vi "test_spline_fft.vi"() -> ()   [LabVIEW 2009]
doc: "Copyright (C) 2009, Stepan A. Baranov\nweb: http://www.OCTLab.org/\nemail: stepan@baranov.su"
uses:
  <vilib>/Analysis/4window.llb/Hanning Window (DBL).vi
  <vilib>/Analysis/NI_AALPro.lvlib
  OCTLib.dll
panel:
  out "error out":errorcluster
  out "Im part":dbl[](array[numeric])
  out "Re part":dbl[](array[numeric])
  out "Phase A-scan":dbl[](array[numeric])
  out "Intensity A-scan":dbl[](array[numeric])
  out "Im":dbl[](array[numeric])
  out "Re":dbl[](array[numeric])
  out "phase":dbl[](array[numeric])
  out "intensity":dbl[](array[numeric])
  out "time for FFT":u32
  in  "RSM_STAT?":bool=TRUE
  in  "stop":bool
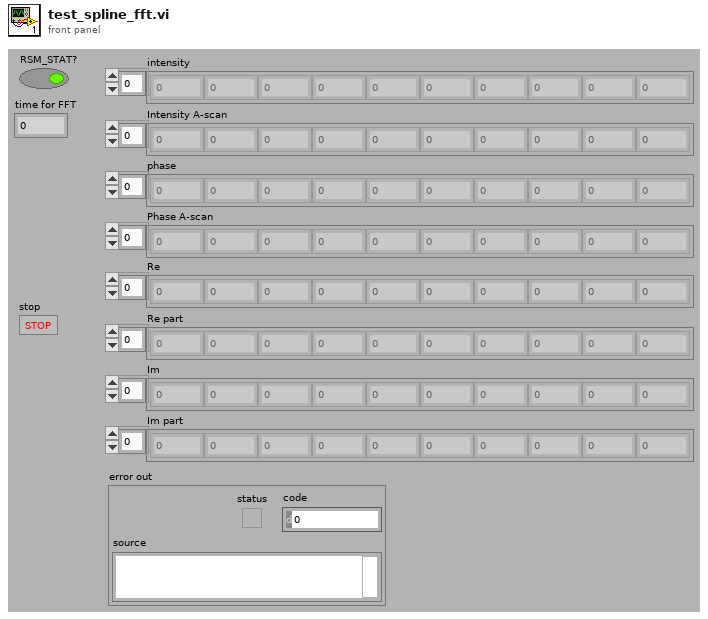
[diagram p1: front panel]
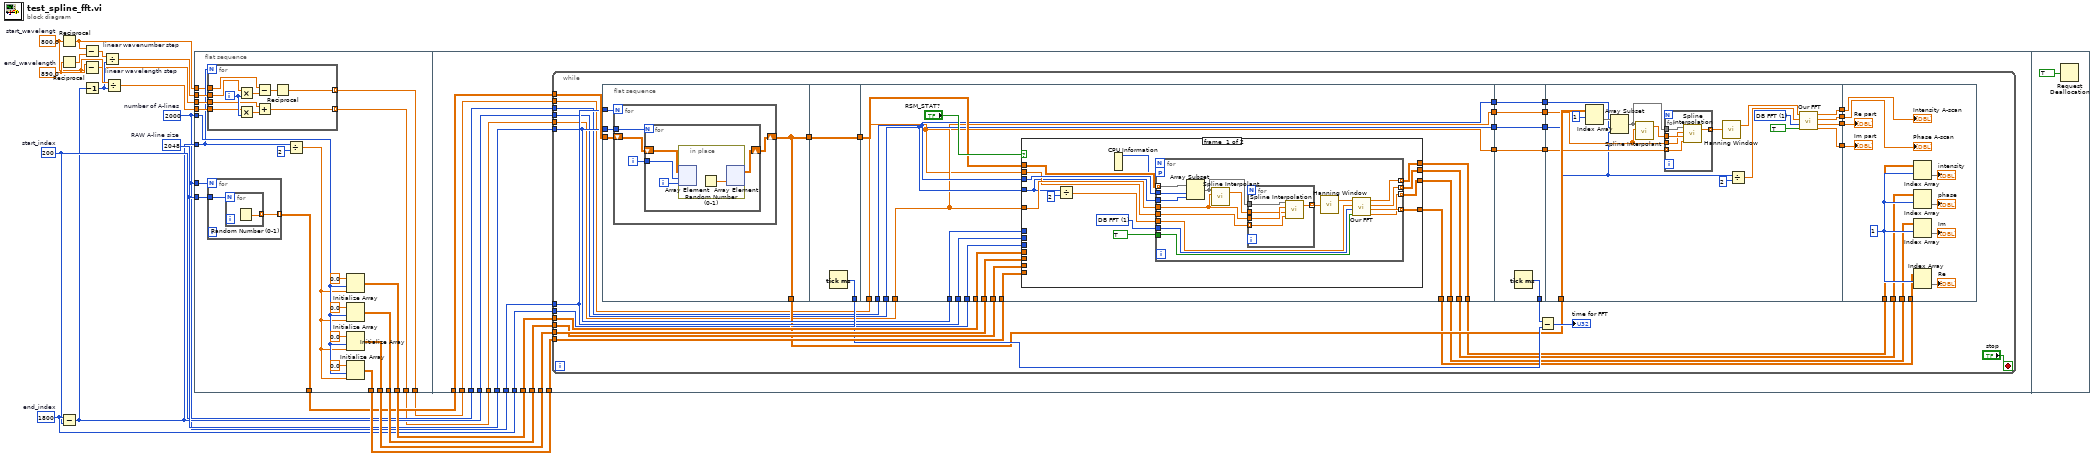
[diagram p0: block diagram]
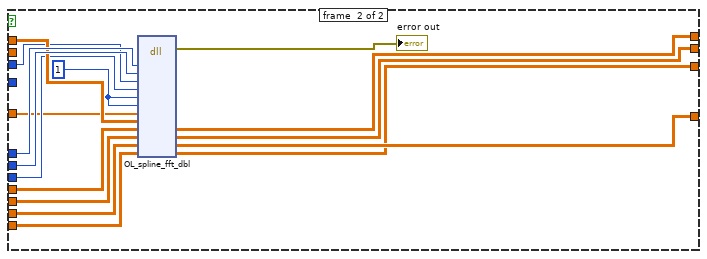
[diagram p2: hidden frame]
diagram:
  w1 = 800.0  # start_wavelengt
  w9 = 890.0  # end_wavelength
  w15 = 1800  # end_index
  w8 = 200  # start_index
  w4 = 2000  # number of A-lines
  w16 = 2048  # RAW A-line size
  n1 = Reciprocal(x=w1) -> (1/x=w2:dbl)
  n2 = Reciprocal(x=w9) -> (1/x=w3:dbl)
  n3 = Subtract(x=w15, y=w8) -> (x-y=w7:i32)
  n4 = Subtract(x=w2, y=w3) -> (x-y=w13:dbl)
  n5 = Subtract(x=w9, y=w1) -> (x-y=w14:dbl)
  n6 = Decrement(x=w7) -> (x-1=w12:i32)
  n7 = Divide "linear wavenumber step"(x=w13, y=w12) -> (x/y=w11:dbl)
  n8 = Divide "linear wavelength step"(x=w14, y=w12) -> (x/y=w10:dbl)
  n9 = flat-sequence {
    tunnel: w16 -> [w42]
    tunnel: w4 -> [w41]
    tunnel: w4 -> [w36]
    tunnel: [w35] -> w21
    tunnel: [w34] -> w20
    tunnel: [w33] -> w19
    tunnel: [w32] -> w18
    tunnel: [w31] -> w17
    tunnel: w7 -> [w26]
    tunnel: w11 -> [w30]
    tunnel: w10 -> [w29]
    tunnel: w1 -> [w28]
    tunnel: [w22] -> w6
    tunnel: [w27] -> w5
    tunnel: w2 -> [w23]
    tunnel: w4 -> [w67]
    tunnel: w16 -> [w66]
    tunnel: w21 -> [w65]
    tunnel: w20 -> [w64]
    tunnel: w19 -> [w63]
    tunnel: w18 -> [w62]
    tunnel: w17 -> [w61]
    tunnel: w8 -> [w60]
    tunnel: w15 -> [w59]
    tunnel: w7 -> [w58]
    tunnel: w6 -> [w57]
    tunnel: w5 -> [w56]
    frame #0 {
      n10 = for {
        N: w26 -> [_]
        tunnel: w30 -> [w52]
        tunnel: [w44] -> w27 mode=indexing
        tunnel: w29 -> [w49]
        tunnel: w28 -> [w48]
        tunnel: [w43] -> w22 mode=indexing
        tunnel: w23 -> [w46]
        i -> [w50]
        n11 = Multiply(x=w52, y=w50) -> (x*y=w51:dbl)
        n12 = Multiply(x=w49, y=w50) -> (x*y=w47:dbl)
        n13 = Subtract(x=w46, y=w51) -> (x-y=w45:dbl)
        n14 = Add(x=w48, y=w47) -> (x+y=w43:dbl)
        n15 = Reciprocal(x=w45) -> (1/x=w44:dbl)
      }
      n16 = for {
        N: w41 -> [_]
        tunnel: [w54] -> w31 mode=indexing
        tunnel: w42 -> [w53]
        n17 = for {
          N: w53 -> [_]
          tunnel: [w55] -> w54 mode=indexing
          n18 = Random Number (0-1)() -> (number: 0 to 1=w55:dbl)
        }
      }
      n19 = Divide(x=w26, y=2) -> (x/y=w24:dbl)
      n20 = Initialize Array(0.0 ("element"), w36, w24) -> (w34:dbl[][])
      n21 = Initialize Array(0.0 ("element"), w36, w24) -> (w33:dbl[][])
      n22 = Initialize Array(0.0 ("element"), w36, w24) -> (w35:dbl[][])
      n23 = Initialize Array(0.0 ("element"), w36, w24) -> (w32:dbl[][])
    }
    frame #1 {
      n24 = while {
        tunnel: w61 -> [w101]
        tunnel: w67 -> [w93]
        tunnel: w66 -> [w92]
        tunnel: w65 -> [w100]
        tunnel: w64 -> [w99]
        tunnel: w63 -> [w98]
        tunnel: w62 -> [w97]
        tunnel: w60 -> [w80]
        tunnel: w59 -> [w79]
        tunnel: w58 -> [w78]
        tunnel: w57 -> [w77]
        tunnel: w56 -> [w76]
        stop <- "stop" stop-if-true
        n25 = flat-sequence {
          tunnel: w101 -> [w106]
          tunnel: w93 -> [w105]
          tunnel: w92 -> [w104]
          tunnel: [w103] -> w91
          tunnel: [w103] -> w81
          tunnel: [w117] -> w96
          tunnel: [w116] -> w82
          tunnel: w81 -> [w116]
          tunnel: w100 -> [w133]
          tunnel: w99 -> [w132]
          tunnel: w98 -> [w131]
          tunnel: w97 -> [w130]
          tunnel: w92 -> [w129]
          tunnel: w93 -> [w128]
          tunnel: [w127] -> w86
          tunnel: [w126] -> w85
          tunnel: [w125] -> w84
          tunnel: [w124] -> w83
          tunnel: w82 -> [w123]
          tunnel: w80 -> [w121]
          tunnel: w79 -> [w122]
          tunnel: w78 -> [w120]
          tunnel: w77 -> [w119]
          tunnel: w76 -> [w118]
          tunnel: [w121] -> w74
          tunnel: [w120] -> w72
          tunnel: [w119] -> w71
          tunnel: [w118] -> w68
          tunnel: [w190] -> w94
          tunnel: [w189] -> w75
          tunnel: w74 -> [w189]
          tunnel: [w188] -> w73
          tunnel: w72 -> [w188]
          tunnel: w71 -> [w187]
          tunnel: [w187] -> w70
          tunnel: [w186] -> w69
          tunnel: w68 -> [w186]
          tunnel: w91 -> [w209]
          tunnel: [w204] -> w90
          tunnel: [w203] -> w89
          tunnel: [w202] -> w88
          tunnel: [w201] -> w87
          tunnel: w75 -> [w198]
          tunnel: w73 -> [w193]
          tunnel: w70 -> [w196]
          tunnel: w69 -> [w195]
          tunnel: w90 -> [w227]
          tunnel: w89 -> [w226]
          tunnel: w88 -> [w225]
          tunnel: w87 -> [w224]
          tunnel: w86 -> [w222]
          tunnel: w85 -> [w220]
          tunnel: w84 -> [w218]
          tunnel: w83 -> [w216]
          frame #0 {
            n26 = for {
              N: w105 -> [_]
              shift-right: [w108] -> w103
              shift-left: w106 -> [w109]
              tunnel: w104 -> [w110]
              i -> [w107]
              n27 = for {
                N: w110 -> [_]
                shift-right: [w111] -> w108
                shift-left: w109 -> [w114]
                tunnel: w107 -> [w113]
                i -> [w112]
                n28 = in-place {
                  n29 = in-place-array #1(w114, w113, w112) -> ()  [unwired: 1 out]
                  n30 = Random Number (0-1)() -> (number: 0 to 1=w115:dbl)
                  n31 = in-place-array #1(w115) -> (w111:dbl[][])  [unwired: 2 out]
                }
              }
            }
          }
          frame #1 {
            n32 = Tick Count (ms)() -> (millisecond timer value=w117:u32)
          }
          frame #2 {
            n33 = case shown="True" "RSM_STAT?" {
              tunnel: w133 -> [_ w182]
              tunnel: w132 -> [_ w185]
              tunnel: w131 -> [_ w184]
              tunnel: w130 -> [_ w183]
              tunnel: w129 -> [_ w181]
              tunnel: w128 -> [_ w180]
              tunnel: w123 -> [w148 w178]
              tunnel: [w144 w177] -> w127
              tunnel: [w143 w176] -> w126
              tunnel: [w142 w175] -> w125
              tunnel: [w141 w174] -> w124
              tunnel: w121 -> [w140 w173]
              tunnel: w122 -> [_ w172]
              tunnel: w120 -> [w137 _]
              tunnel: w119 -> [w139 w170]
              tunnel: w118 -> [w138 _]
              frame #0 {
                w145 = 1 items=["LINEAR FFT", "DB FFT"] ("A-scan type")
                n34 = Divide(x=w137, y=2) -> (x/y=w135:dbl)
                n35 = CPU Information() -> (4:w147:i32)  [unwired: 3 out]
                n36 = for {
                  workers-P: w147 -> [_]
                  tunnel: [w163] -> w144 mode=indexing
                  tunnel: [w162] -> w143 mode=indexing
                  tunnel: [w161] -> w142 mode=indexing
                  tunnel: [w160] -> w141 mode=indexing
                  tunnel: w148 -> [w157] mode=indexing
                  tunnel: TRUE ("need phase?") -> [w159]
                  tunnel: w145 -> [w158]
                  tunnel: w140 -> [w156]
                  tunnel: w137 -> [w155]
                  tunnel: w139 -> [w152]
                  tunnel: w138 -> [w154]
                  tunnel: w135 -> [w149]
                  n37 = Array Subset(array=w157, index=w156, length=w155) -> (w153:dbl[])
                  n38 = call <vilib>:"Spline Interpolant.vi"("X"=w152, "Y"=w153) -> ("Interpolant"=w151:dbl[])  [unwired: 2 in, 1 out]
                  n39 = for {
                    tunnel: w154 -> [w166] mode=indexing
                    tunnel: w153 -> [w169]
                    tunnel: w152 -> [w168]
                    tunnel: w151 -> [w167]
                    tunnel: [w165] -> w150 mode=indexing
                    n40 = call <vilib>:"Spline Interpolation.vi"("x value"=w166, "Interpolant"=w167, "X"=w168, "Y"=w169) -> ("interpolation value"=w165:dbl)  [unwired: 1 out]
                  }
                  n41 = call-poly <vilib>:"Hanning Window.vi"("X"=w150) -> ("Windowed X"=w164:dbl[])  [unwired: 1 out]
                  n42 = call "Our FFT.vi"("need phase?"=w159, "A-scan type"=w158, "FFT A-scan size"=w149, "RAW A-line"=w164) -> ("Im part"=w160:dbl[], "Re part"=w161:dbl[], "Phase A-scan"=w162:dbl[], "Intensity A-scan"=w163:dbl[])
                }
              }
              frame #1 {
                w179 = i8 1 ("hanning_flag")
                n43 = dll-call lib="OCTLib.dll" fn="OL_spline_fft_dbl"("width"=w181, "height"=w180, "start_index"=w173, "end_index"=w172, "hanning_flag"=w179, "log10_flag"=w179, "spectrum"=w170, "input"=w178, "intensity"=w185, "phase"=w184, "Re"=w182, "Im"=w183) -> (error out=→"error out":errorcluster, "intensity"=w177:dbl[][], "phase"=w176:dbl[][], "Re"=w175:dbl[][], "Im"=w174:dbl[][])  [unwired: 12 in, 1 out]
              }
            }
          }
          frame #3 {
            n44 = Tick Count (ms)() -> (millisecond timer value=w190:u32)
          }
          frame #4 {
            w206 = 1 items=["LINEAR FFT", "DB FFT"] ("A-scan type")
            n45 = Index Array(array=w209, index (row)=1) -> (element=w199:dbl[])  [unwired: 1 in]
            n46 = Array Subset(array=w199, index=w198, length=w193) -> (w197:dbl[])
            n47 = call <vilib>:"Spline Interpolant.vi"("X"=w196, "Y"=w197) -> ("Interpolant"=w200:dbl[])  [unwired: 2 in, 1 out]
            n48 = for {
              tunnel: w200 -> [w214]
              tunnel: w197 -> [w213]
              tunnel: w196 -> [w212]
              tunnel: w195 -> [w211] mode=indexing
              tunnel: [w210] -> w194 mode=indexing
              n49 = call <vilib>:"Spline Interpolation.vi"("x value"=w211, "Interpolant"=w214, "X"=w212, "Y"=w213) -> ("interpolation value"=w210:dbl)  [unwired: 1 out]
            }
            n50 = call-poly <vilib>:"Hanning Window.vi"("X"=w194) -> ("Windowed X"=w207:dbl[])  [unwired: 1 out]
            n51 = Divide(x=w193, y=2) -> (x/y=w191:dbl)
            n52 = call "Our FFT.vi"("need phase?"=TRUE, "A-scan type"=w206, "FFT A-scan size"=w191, "RAW A-line"=w207) -> ("Im part"=w201:dbl[], "Re part"=w202:dbl[], "Phase A-scan"=w203:dbl[], "Intensity A-scan"=w204:dbl[])
          }
          frame #5 {
            w223 = 1 ("index (row)")
            n53 = Index Array(array=w222, index (row)=w223) -> (element=→"intensity":dbl[])  [unwired: 1 in]
            n54 = Index Array(array=w220, index (row)=w223) -> (element=→"phase":dbl[])  [unwired: 1 in]
            n55 = Index Array(array=w216, index (row)=w223) -> (element=→"Im":dbl[])  [unwired: 1 in]
            n56 = Index Array(array=w218, index (row)=w223) -> (element=→"Re":dbl[])  [unwired: 1 in]
            "Intensity A-scan" <- w227
            "Phase A-scan" <- w226
            "Re part" <- w225
            "Im part" <- w224
          }
        }
        n57 = Subtract(x=w94, y=w96) -> (x-y=→"time for FFT":u32)
      }
    }
    frame #2 {
      n58 = Request Deallocation(TRUE ("flag")) -> ()
    }
  }
